vi "读取database数据.vi"(10 "table输入":string(combo), 11 "起始时间":string) -> (0 "error out":errorcluster, 3 "data":string[][](table))   [LabVIEW 2016]
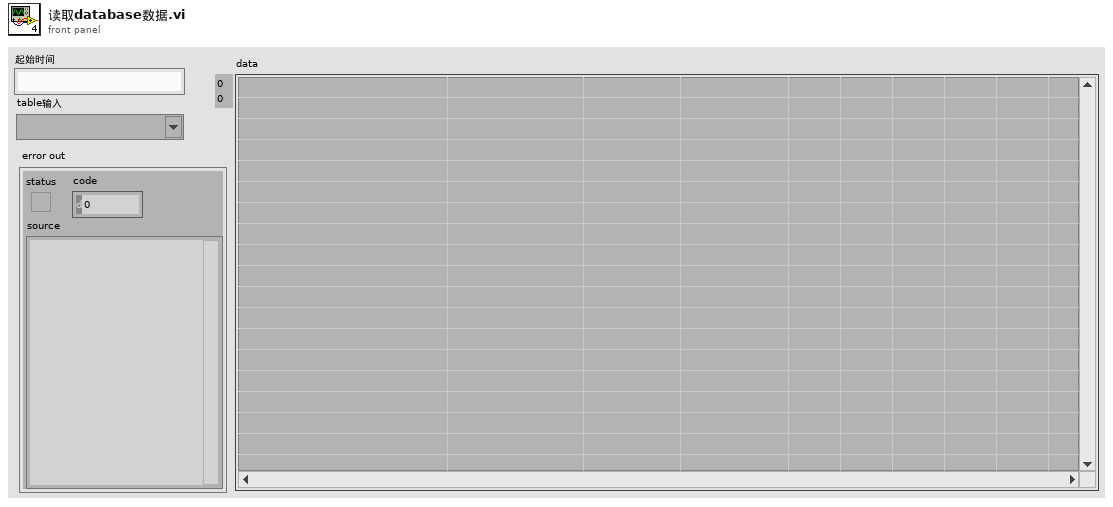
[diagram p1: front panel]
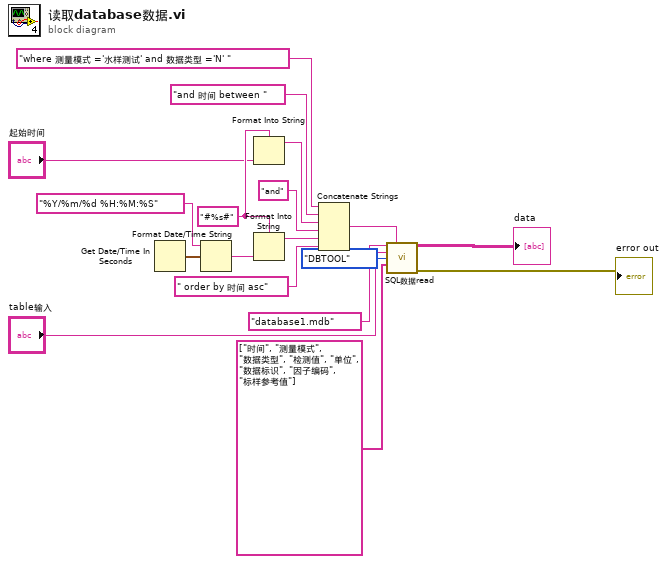
[diagram p0: block diagram]
diagram:
  w10 = "#%s#" ("初始字符串")
  n1 = Get Date/Time In Seconds() -> (seconds since 1Jan1904=w13:timestamp)
  n2 = Format Date/Time String(time format string (%c)="%Y/%m/%d %H:%M:%S" ("时间格式字符串(%c)"), seconds (now)=w13) -> (date/time string=w11:string)  [unwired: 1 in]
  n3 = Format Into String(format string=w10, "起始时间") -> (resulting string=w9:string)  [unwired: 2 in, 1 out]
  n4 = Format Into String(format string=w10, w11) -> (resulting string=w14:string)  [unwired: 2 in, 1 out]
  n5 = Concatenate Strings("where 测量模式 ='水样测试' and 数据类型 ='N' " ("condition"), "and 时间 between ", w9, "and" ("字符串"), w14, " order by 时间 asc" ("字符串")) -> (w7:string)
  n6 = call "SQL数据read.vi"("database"="database1.mdb", "condition"=w7, "table输入"="table输入", "枚举"=enum16{"DBTOOL", "SQLquery"}."DBTOOL", "columns"=string[] ["时间", "测量模式", "数据类型", "检测值", "单位", "数据标识", "因子编码", "标样参考值"]) -> ("data"=→"data":string[][], "error out"=→"error out":errorcluster)  [unwired: 8 in, 1 out]
